vi "setDefaultPath.vi"(8 "error in (no error)":errorcluster, 10 "Default Path":path, 11 "settingsViewer.lvclass in":refnum<class "settingsViewer.lvclass">) -> (0 "error out":errorcluster, 3 "settingsViewer.lvclass out":refnum<class "settingsViewer.lvclass">)   [LabVIEW 2009, in "Views.lvlib" / "SettingsViewer.lvclass"]
uses:
  settingsViewer.lvclass
  settingsViewer.lvclass/settingsViewer.ctl
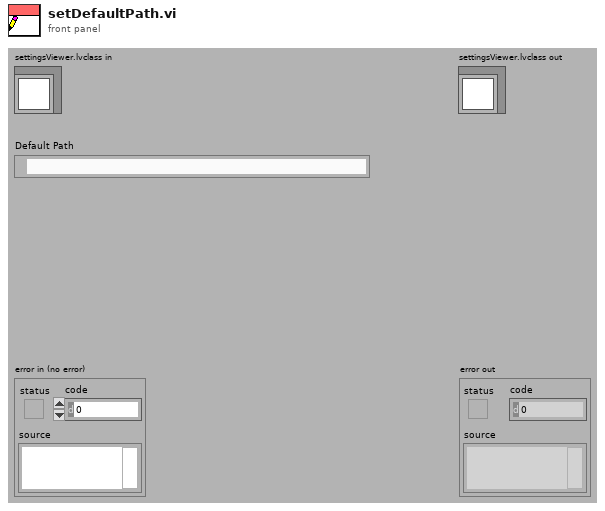
[diagram p1: front panel]
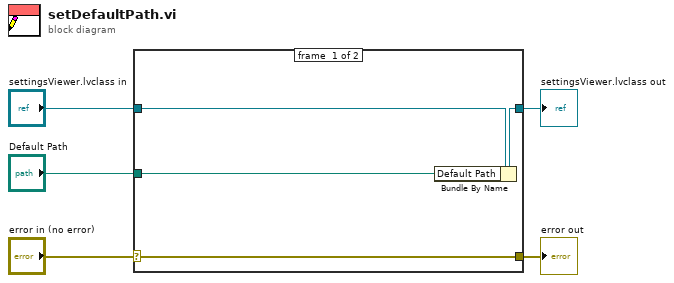
[diagram p0: block diagram]
diagram:
  n1 = case shown="No Error" "error in (no error)" {
    selector: "error in (no error)" -> [w9 w10]
    tunnel: [w9 w10] -> w4
    tunnel: [w7 w11] -> w2
    tunnel: "settingsViewer.lvclass in" -> [w8 w11]
    tunnel: "Default Path" -> [w6 _]
    frame #0 {
      n2 = Bundle By Name(cluster=w8, "Default Path"=w6) -> (w7:refnum<class "settingsViewer.lvclass">)
    }
    frame #1 {
    }
  }
  "error out" <- w4
  "settingsViewer.lvclass out" <- w2
